vi "SendHistoryResults.vi"(8 "error in (no error)":errorcluster, 11 "TopLevel in":refnum<class "TopLevel.lvclass">) -> (0 "error out":errorcluster, 3 "TopLevel out":refnum<class "TopLevel.lvclass">)   [LabVIEW 2021, in "TopLevel.lvlib" / "TopLevel.lvclass"]
uses:
  TopLevel.lvclass
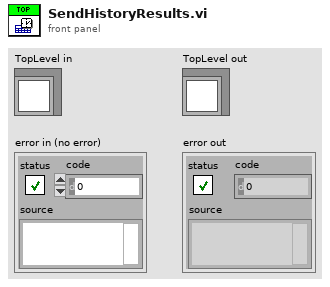
[diagram p1: front panel]
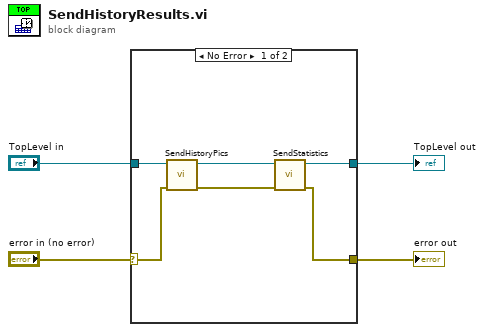
[diagram p0: block diagram]
diagram:
  n1 = case shown="No Error" "error in (no error)" {
    selector: "error in (no error)" -> [w7 w12]
    tunnel: [w9 w12] -> w3
    tunnel: [w10 w11] -> w1
    tunnel: "TopLevel in" -> [w8 w11]
    frame No Error {
      n2 = call "SendHistoryPics.vi"("error in (no error)"=w7, "TopLevel in"=w8) -> ("error out"=w5:errorcluster, "TopLevel out"=w6:refnum<class "TopLevel.lvclass">)  [unwired: 8 in]
      n3 = call "SendStatistics.vi"("error in (no error)"=w5, "TopLevel in"=w6) -> ("error out"=w9:errorcluster, "TopLevel out"=w10:refnum<class "TopLevel.lvclass">)  [unwired: 8 in]
    }
    frame Error {
    }
  }
  "error out" <- w3
  "TopLevel out" <- w1
